vi "LRC-8.vi"(11 "data":u8[](array[numeric])) -> (3 "LRC-8":u8)   [LabVIEW 2020, in "SubVIs.lvlib" / "ASCII Data Unit.lvclass"]
doc: "Performs a longitudinal redundancy check which generates an 8-bit number. This must be converted into ASCII for the ASCII ADU."
uses:
  <vilib>/Modbus/subvis/Transmission Data Unit (ADU)/ASCII Data Unit/ASCII Data Unit.lvclass
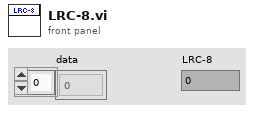
[diagram p1: front panel]
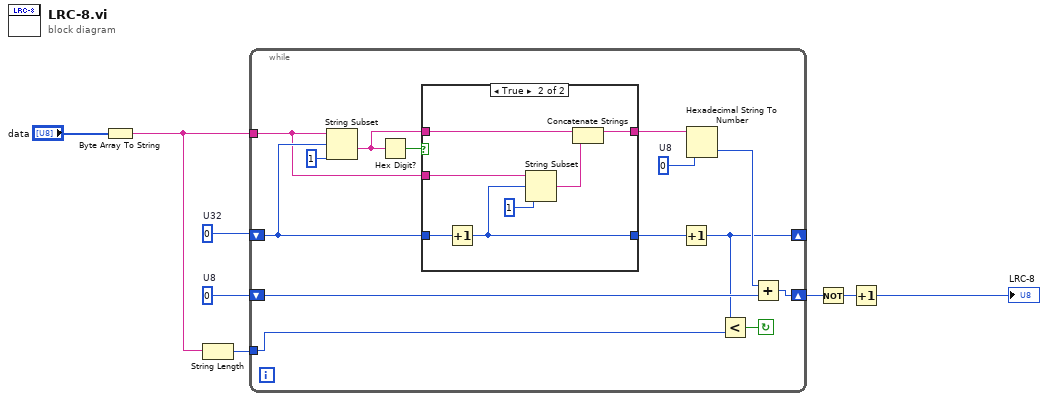
[diagram p0: block diagram]
diagram:
  w8 = u32 0  # U32
  w7 = u8 0  # U8
  n1 = Byte Array To String(unsigned byte array="data") -> (string=w2:string)
  n2 = String Length(string=w2) -> (length=w6:i32)
  n3 = while {
    tunnel: w2 -> [w17]
    tunnel: w6 -> [w10]
    shift-left: w7 -> [w14]
    shift-right: [w13] -> w5
    shift-left: w8 -> [w21]
    shift-right: [w9] -> _
    stop <- w11 continue-if-true
    w16 = u8 0  # U8
    n4 = String Subset(string=w17, offset (0)=w21, length (rest)=1) -> (substring=w18:string)
    n5 = Hex Digit?(1:w18) -> (0:w19:bool)
    n6 = case shown="True" w19 {
      tunnel: w21 -> [w23 w31]
      tunnel: [w23 w29] -> w20
      tunnel: w18 -> [w24 w27]
      tunnel: w17 -> [_ w28]
      tunnel: [w24 w25] -> w15
      frame False {
      }
      frame True {
        n7 = Increment(x=w31) -> (x+1=w29:u32)
        n8 = String Subset(string=w28, offset (0)=w29, length (rest)=1) -> (substring=w26:string)
        n9 = Concatenate Strings(w27, w26) -> (w25:string)
      }
    }
    n10 = Increment(x=w20) -> (x+1=w9:u32)
    n11 = Hexadecimal String To Number(string=w15, default (0uL)=w16) -> (number=w12:u8)  [unwired: 2 out]
    n12 = Less?(x=w9, y=w10) -> (x < y?=w11:bool)
    n13 = Add(x=w12, y=w14) -> (x+y=w13:u8)
  }
  n14 = Not(x=w5) -> (.not. x?=w4:u8)
  n15 = Increment(x=w4) -> (x+1=→"LRC-8":u8)
